vi "Encoding Message from GUI.vi"(8 "Data":string, 9 "Message":string, 10 "uS/GD ID":string, 11 "uService Template in":refnum<class "TCP Writer.lvclass">) -> (2 "Variant":variant, 3 "uService Template out":refnum<class "TCP Writer.lvclass">)   [LabVIEW 2026, in "TALOS.lvlib" / "TCP Writer.lvlib" / "TCP Writer.lvclass"]
uses:
  TCP Writer.lvclass
  TCP Message Internal Composition.ctl
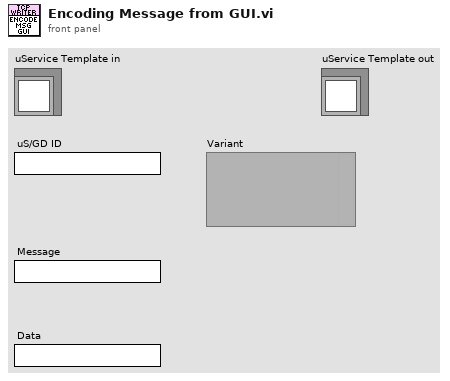
[diagram p1: front panel]
types:
  T1 = typedef "TALOS.lvlib/TCP Writer.lvlib/TCP Writer.lvclass/TCP Message Internal Composition.ctl" = cluster{"uS/GD ID":string, "Message":string, "Data":variant}
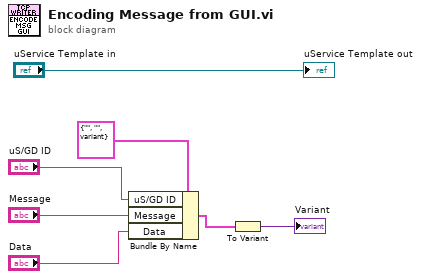
[diagram p0: block diagram]
diagram:
  n1 = Bundle By Name(cluster=T1 {"uS/GD ID"="", "Message"="", "Data"=variant}, "uS/GD ID"="uS/GD ID", "Message"="Message", "Data"="Data") -> (w4:T1)
  n2 = To Variant(anything=w4) -> (Variant=→"Variant":variant)
  "uService Template out" <- "uService Template in"
